vi "mod T params.vi"(0 "Set T params":bool, 11 "error in (no error)":errorcluster) -> (15 "error out":errorcluster)   [LabVIEW 2019]
doc: "This is a Bug C(T) subVI.\n\nIt is a shell for a popup that allows the user to modify the temp control parameters from the monitor loop.\n\nPaul K Dixon\nP3600\nCSUSB Physics"
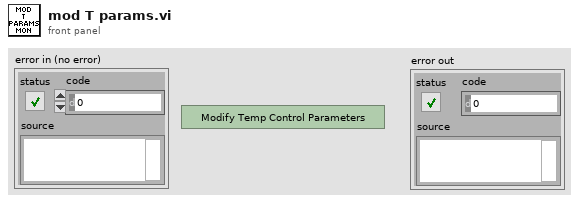
[diagram p1: front panel]
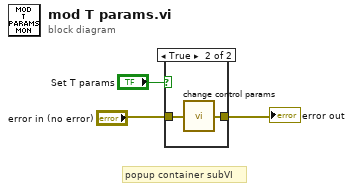
[diagram p0: block diagram]
diagram:
  # "popup container subVI"
  n1 = case shown="True" "Set T params" {
    tunnel: "error in (no error)" -> [w4 w6]
    tunnel: [w4 w5] -> w1
    frame False {
    }
    frame True {
      n2 = call "change control params.vi"("exp exec in"=w6) -> ("exp exec in"=w5:errorcluster)  [unwired: 14 in]
    }
  }
  "error out" <- w1
